vi "SetTriggerHW.vi"(8 "error in (no error)":errorcluster, 11 "BME_DG_Base in":refnum<class "BME_DG_Base.lvclass">) -> (0 "error out":errorcluster, 3 "BME_DG_Base out":refnum<class "BME_DG_Base.lvclass">)   [LabVIEW 2009, in "BME_DG_Base.lvclass"]
uses:
  BME_DG_Base.lvclass
  Applied Energetics Stuff/SubVI/Settings.ctl
  BME_DG_Base.lvclass/BME_DG_Base.ctl
panel:
  in  "Settings":T1={"T Delay (µs)"=0.0, "T Set Back"=1.0, "T Triggers"=1, "T Active"=TRUE, "T Polarity"=TRUE, "T Term"=FALSE, "T Drive"=FALSE, "A Delay (µs)"=3.0, "A Set Back"=1.0, "A Triggers"=1, "A Active"=TRUE, "A Polarity"=TRUE, "A Term"=FALSE, "A Drive"=FALSE, "B Delay (µs)"=4.0, "B Set Back"=1.0, "B Triggers"=1, "B Active"=TRUE, "B Polarity"=TRUE, "B Term"=FALSE, "B Drive"=FALSE, "Gate A*B"=FALSE, "Output\nLevel"=1, "Trigger\nTerminate"=TRUE, "Clock\nEnable"=TRUE, "Internal\nClock (µs)"=1.0, "Trigger\nLevel"=10.0, "Stop\nTrigger"=1, "Ocillator\nDivide By"=1, "Clock Source"=1, "Gate Divider"=1, "Positive\nGate"=TRUE, "Trigger\nSource"=FALSE, "Internal\nArming"=FALSE, "Software\nTrigger"=TRUE, "Trigger\nSlope"=FALSE, "Stop on\nPreset"=TRUE, "Trigger\nOperation"=TRUE, "Trigger\nEnable"=TRUE} {"B Set Back" min=0.0 format="%.3f"; "A Set Back" min=0.0 format="%.3f"; "T Set Back" min=0.0 format="%.3f"; "Clock Source" items=["Internal Oscillator"=1, "External Trigger"=2, "Trigger & Oscillator"=3, "Master Slave Bus"=4]; "Trigger\nLevel" min=0.0 format="%.3f"; "Output\nLevel" items=["TTL"=1, "NIM"=2, "ECL"=3]; "Internal\nClock (µs)" min=0.0 format="%.4f"; "B Delay (µs)" min=0.0 format="%.3f"; "A Delay (µs)" min=0.0 format="%.3f"; "T Delay (µs)" min=0.0 format="%.3f"}
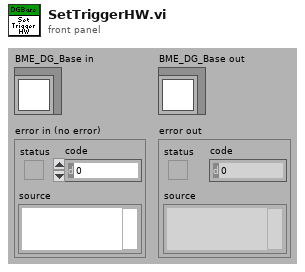
[diagram p1: front panel]
types:
  T1 = typedef "Settings.ctl" = cluster{"T Delay (µs)":dbl, "T Set Back":dbl, "T Triggers":u16, "T Active":bool, "T Polarity":bool, "T Term":bool, "T Drive":bool, "A Delay (µs)":dbl, "A Set Back":dbl, "A Triggers":u16, "A Active":bool, "A Polarity":bool, "A Term":bool, "A Drive":bool, "B Delay (µs)":dbl, "B Set Back":dbl, "B Triggers":u16, "B Active":bool, "B Polarity":bool, "B Term":bool, "B Drive":bool, "Gate A*B":bool, "Output\nLevel":u32, "Trigger\nTerminate":bool, "Clock\nEnable":bool, "Internal\nClock (µs)":dbl, "Trigger\nLevel":dbl, "Stop\nTrigger":u32, "Ocillator\nDivide By":u16, "Clock Source":u32, "Gate Divider":u32, "Positive\nGate":bool, "Trigger\nSource":bool, "Internal\nArming":bool, "Software\nTrigger":bool, "Trigger\nSlope":bool, "Stop on\nPreset":bool, "Trigger\nOperation":bool, "Trigger\nEnable":bool}
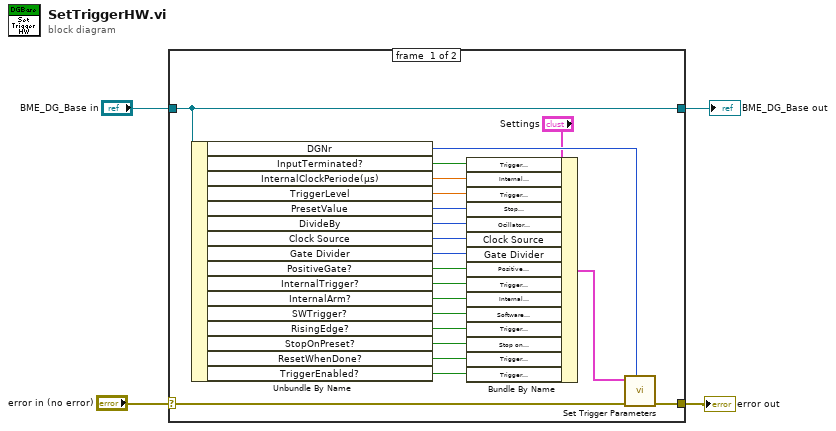
[diagram p0: block diagram]
diagram:
  n1 = case shown="No Error" "error in (no error)" {
    selector: "error in (no error)" -> [w24 w27]
    tunnel: [w23 w27] -> w3
    tunnel: [w25 w26] -> w1
    tunnel: "BME_DG_Base in" -> [w25 w26]
    frame #0 {
      n2 = Unbundle By Name(w25) -> ("DGNr"=w22:i32, "InputTerminated?"=w19:bool, "InternalClockPeriode(µs)"=w18:dbl, "TriggerLevel"=w17:dbl, "PresetValue"=w16:i32, "DivideBy"=w15:i32, "Clock Source"=w14:u32, "Gate Divider"=w13:i32, "PositiveGate?"=w12:bool, "InternalTrigger?"=w11:bool, "InternalArm?"=w10:bool, "SWTrigger?"=w9:bool, "RisingEdge?"=w8:bool, "StopOnPreset?"=w7:bool, "ResetWhenDone?"=w6:bool, "TriggerEnabled?"=w5:bool)
      n3 = Bundle By Name(cluster="Settings", "Trigger\nTerminate"=w19, "Internal\nClock (µs)"=w18, "Trigger\nLevel"=w17, "Stop\nTrigger"=w16, "Ocillator\nDivide By"=w15, "Clock Source"=w14, "Gate Divider"=w13, "Positive\nGate"=w12, "Trigger\nSource"=w11, "Internal\nArming"=w10, "Software\nTrigger"=w9, "Trigger\nSlope"=w8, "Stop on\nPreset"=w7, "Trigger\nOperation"=w6, "Trigger\nEnable"=w5) -> (w20:T1)
      n4 = call "Set Trigger Parameters.vi"("DG Number"=w22, "error in (no error)"=w24, "Settings"=w20) -> ("error out"=w23:errorcluster)  [unwired: 8 in]
    }
    frame #1 {
    }
  }
  "error out" <- w3
  "BME_DG_Base out" <- w1
